vi "TAGs_AURAwheel_inycom.vi"(4 "Plataformas?":bool, 6 "TAGs LR6":string[](array[string]), 7 "TAGs":string[](array[string]), 8 "it-read-LR6":i32[](array[numeric]), 9 "it-LR6":i32, 10 "Ejes_convoy":i32, 11 "Nº Ejes":i32[](array[numeric])) -> (3 "TAGS_AURA":string[][](array[string]))   [LabVIEW 2015]
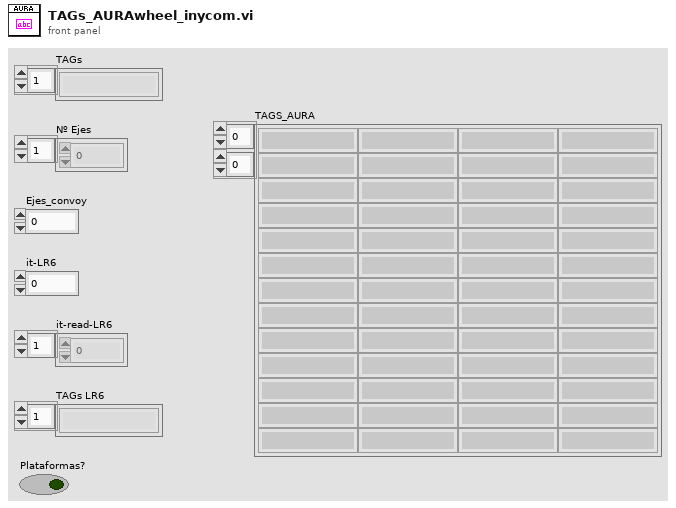
[diagram p1: front panel]
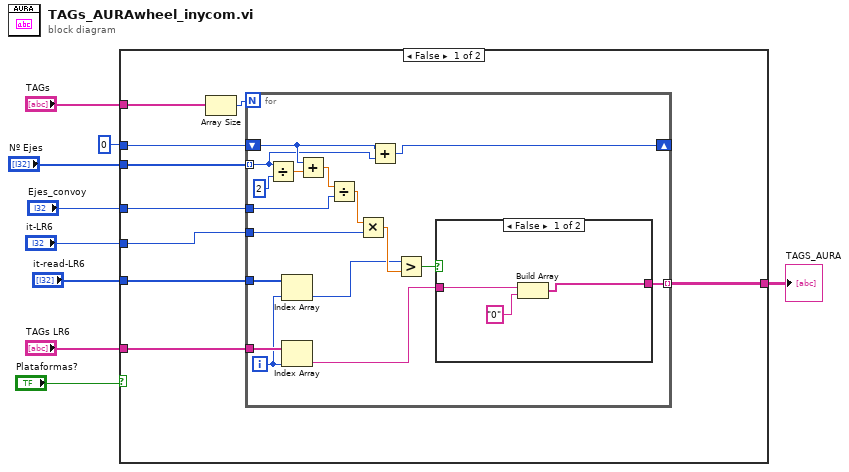
[diagram p0: block diagram]
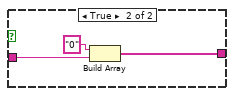
[diagram p2: hidden frame]
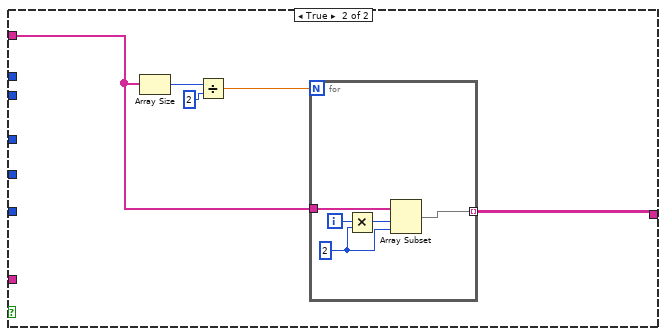
[diagram p3: hidden frame]
diagram:
  n1 = case shown="False" "Plataformas?" {
    tunnel: "TAGs LR6" -> [w17 _]
    tunnel: "it-LR6" -> [w13 _]
    tunnel: "it-read-LR6" -> [w16 _]
    tunnel: "Nº Ejes" -> [w15 _]
    tunnel: "Ejes_convoy" -> [w14 _]
    tunnel: "TAGs" -> [w12 w43]
    tunnel: [w11 w42] -> w8
    tunnel: 0 -> [w10 _]
    frame False {
      n2 = Array Size(array=w12) -> (size(s)=w18:i32)
      n3 = for {
        N: w18 -> [_]
        tunnel: w17 -> [w35]
        tunnel: w16 -> [w34]
        tunnel: w15 -> [w20] mode=indexing
        tunnel: w14 -> [w31]
        tunnel: w13 -> [w29]
        tunnel: [w24] -> w11 mode=indexing
        shift-right: [w19] -> _
        shift-left: w10 -> [w21]
        i -> [w33]
        n4 = Divide(x=w20, y=2) -> (x/y=w23:dbl)
        n5 = Index Array(array=w34, index=w33) -> (element=w27:i32)
        n6 = Index Array(array=w35, index=w33) -> (element=w25:string)
        n7 = Add(x=w21, y=w23) -> (x+y=w22:dbl)
        n8 = Divide(x=w22, y=w31) -> (x/y=w30:dbl)
        n9 = Multiply(x=w30, y=w29) -> (x*y=w28:dbl)
        n10 = Add(x=w21, y=w20) -> (x+y=w19:i32)
        n11 = Greater?(x=w27, y=w28) -> (0:w26:bool)
        n12 = case shown="False" w26 {
          tunnel: w25 -> [w37 w41]
          tunnel: [w36 w39] -> w24
          frame False {
            n13 = Build Array(w37, "0" ("element")) -> (w36:string[])
          }
          frame True {
            n14 = Build Array("0" ("element"), w41) -> (w39:string[])
          }
        }
      }
    }
    frame True {
      n15 = Array Size(array=w43) -> (size(s)=w46:i32)
      n16 = Divide(x=w46, y=2) -> (x/y=w44:dbl)
      n17 = for {
        N: w44 -> [_]
        tunnel: w43 -> [w51]
        tunnel: [w47] -> w42 mode=indexing
        i -> [w50]
        w48 = 2 ("y")
        n18 = Multiply(x=w50, y=w48) -> (x*y=w49:i32)
        n19 = Array Subset(array=w51, index=w49, length=w48) -> (w47:string[])
      }
    }
  }
  "TAGS_AURA" <- w8
